vi "Update Devices Menu.vi"(8 "error in":errorcluster) -> (0 "error out":errorcluster, 1 "New Menu":string[](array[string]))   [LabVIEW 2024, in "Data Base.lvlib"]
uses:
  Data Base.lvlib
  Support/General Type Defs/Global Data.vi
  Support/General Type Defs/General Type Defs.lvlib
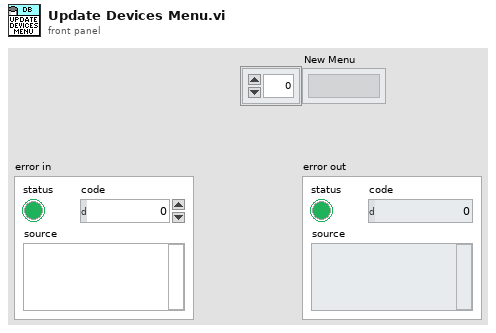
[diagram p1: front panel]
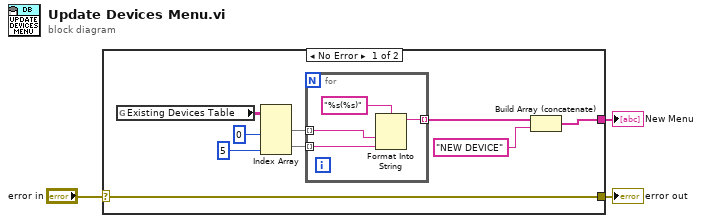
[diagram p0: block diagram]
diagram:
  n1 = case shown="No Error" "error in" {
    selector: "error in" -> [w6 w17]
    tunnel: [w5 _] -> w3
    tunnel: [w6 w17] -> w1
    frame No Error {
      n2 = global read "Global Data.vi" "Existing Devices Table"() -> (w12:string[][])
      n3 = Index Array(array=w12, index (col) #1=0 ("index (col)"), index (col) #2=5 ("index (col)")) -> (element #1=w9:string[], element #2=w8:string[])  [unwired: 2 in]
      n4 = for {
        tunnel: w9 -> [w15] mode=indexing
        tunnel: w8 -> [w14] mode=indexing
        tunnel: [w13] -> w7 mode=indexing
        n5 = Format Into String(format string="%s(%s)", w15, w14) -> (resulting string=w13:string)  [unwired: 2 in, 1 out]
      }
      n6 = Build Array (concatenate)(w7, "NEW DEVICE" ("format string")) -> (w5:string[])
    }
    frame Error {
    }
  }
  "error out" <- w1
  "New Menu" <- w3
